vi "仪器参数设置.vi"(11 "仪器参数设置输入":T1(array[cluster])) -> (2 "确定":bool, 3 "仪器参数设置输出":T1(array[cluster]))   [LabVIEW 2016, in "斯坦道多参数.lvlib"]
uses:
  <vilib>/Utility/miscctls.llb/LVPointTypeDef.ctl
panel:
  in  "多参数":T2(ring)
  in  "标样校准时间":timestamp
  in  "二次多项式系数":dbl
  in  "线性相关系数":dbl
  in  "测量信号值":dbl
  in  "测量检出限":dbl
  in  "曲线斜率":dbl
  in  "曲线截距":dbl
  in  "空白校准时间":timestamp
  in  "消解时长":dbl
  in  "消解温度":dbl
  in  "测量间隔":dbl
  in  "测量精度":dbl
  in  "测量量程":dbl
  in  "取消":bool
  in  "确定":bool
  # "仪器参数设置"
  # "多参数"
  # "监测参数"
  # "黑色框参数需要手动输入\n灰色框参数自动读取不需要手动输入"
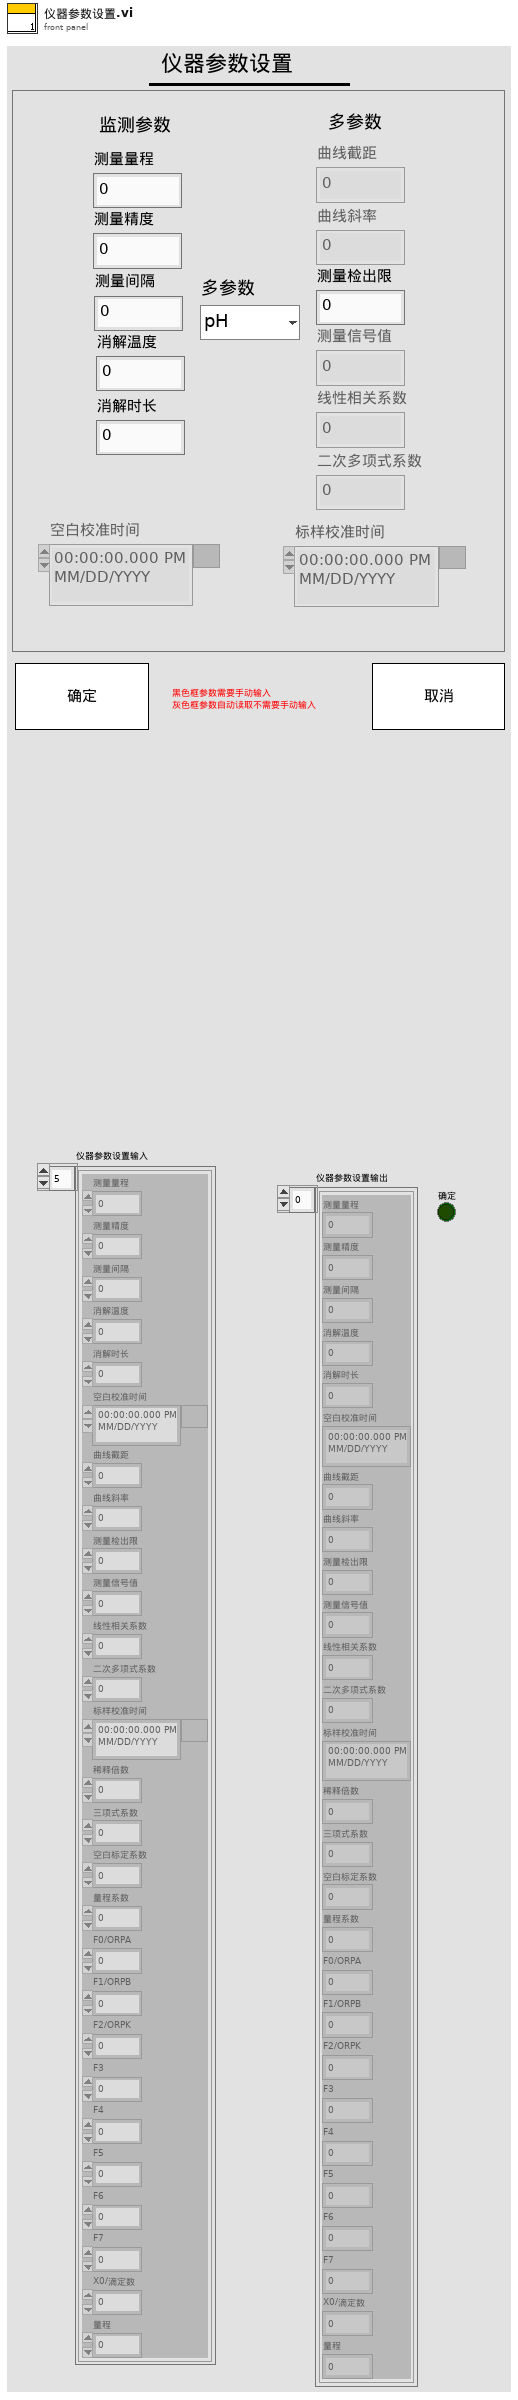
[diagram p1: front panel]
types:
  T1 = cluster{"测量量程":dbl, "测量精度":dbl, "测量间隔":dbl, "消解温度":dbl, "消解时长":dbl, "空白校准时间":timestamp, "曲线截距":dbl, "曲线斜率":dbl, "测量检出限":dbl, "测量信号值":dbl, "线性相关系数":dbl, "二次多项式系数":dbl, "标样校准时间":timestamp, "稀释倍数":dbl, "三项式系数":dbl, "空白标定系数":dbl, "量程系数":dbl, "F0/ORPA":dbl, "F1/ORPB":dbl, "F2/ORPK":dbl, "F3":dbl, "F4":dbl, "F5":dbl, "F6":dbl, "F7":dbl, "X0/滴定数":dbl, "量程":dbl}[]
  T2 = enum16{"pH", "水温", "电导率", "溶解氧", "浊度", "叶绿素", "藻密度", "ORP"}
  T3 = typedef "LVPointTypeDef.ctl" = cluster{"Horizontal":i16, "Vertical":i16}
  T4 = cluster{"测量量程":dbl, "测量精度":dbl, "测量间隔":dbl, "消解温度":dbl, "消解时长":dbl, "空白校准时间":timestamp, "曲线截距":dbl, "曲线斜率":dbl, "测量检出限":dbl, "测量信号值":dbl, "线性相关系数":dbl, "二次多项式系数":dbl, "标样校准时间":timestamp, "稀释倍数":dbl, "三项式系数":dbl, "空白标定系数":dbl, "量程系数":dbl, "F0/ORPA":dbl, "F1/ORPB":dbl, "F2/ORPK":dbl, "F3":dbl, "F4":dbl, "F5":dbl, "F6":dbl, "F7":dbl, "X0/滴定数":dbl, "量程":dbl}
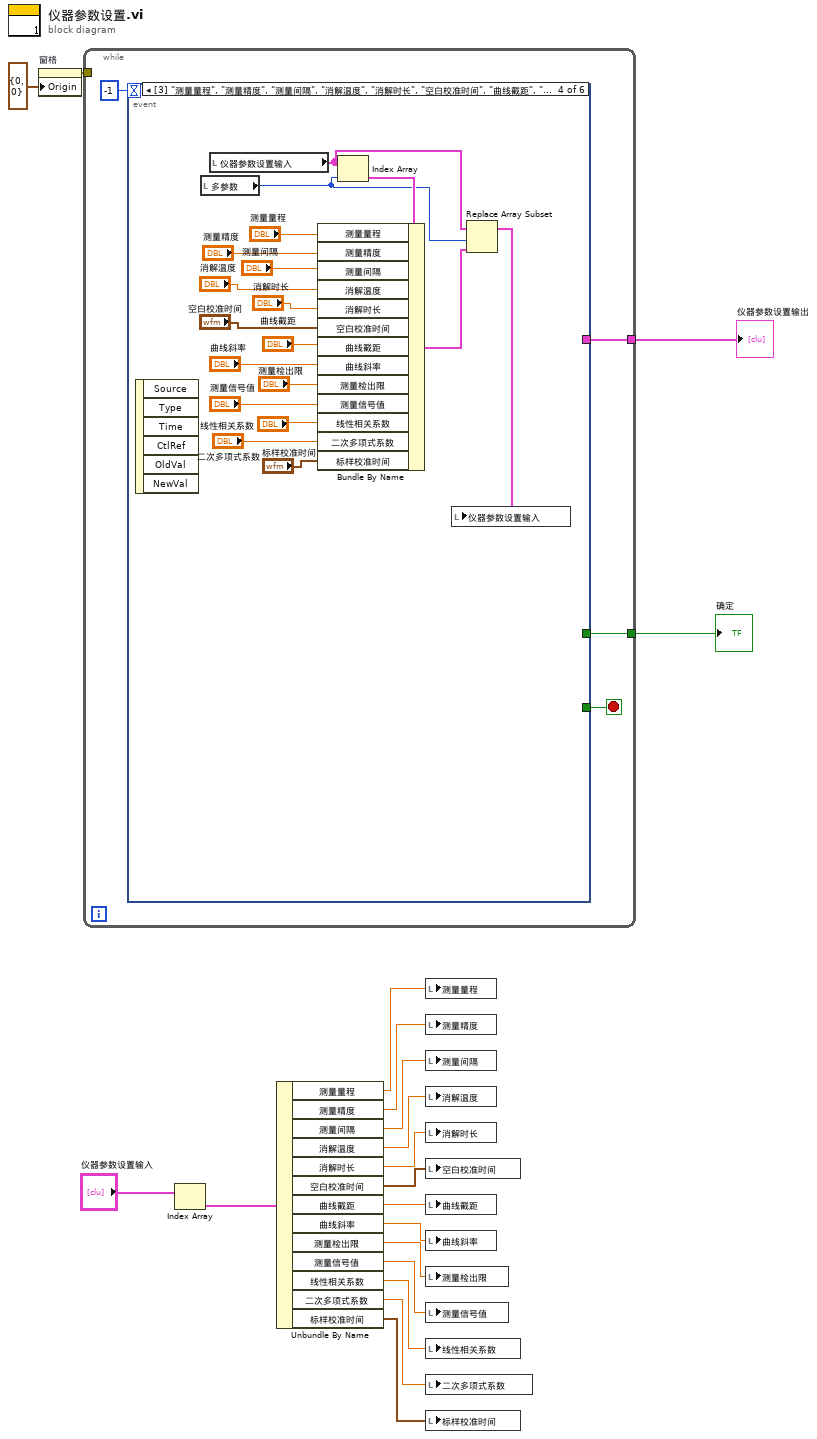
[diagram p0: block diagram]
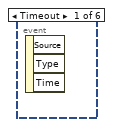
[diagram p2: hidden frame]
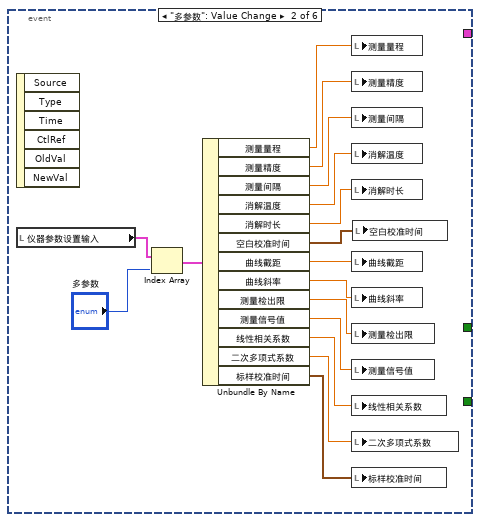
[diagram p3: hidden frame]
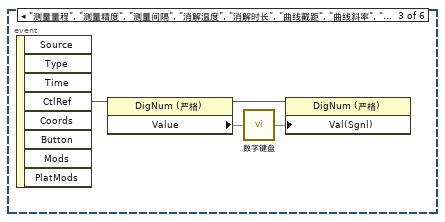
[diagram p4: hidden frame]
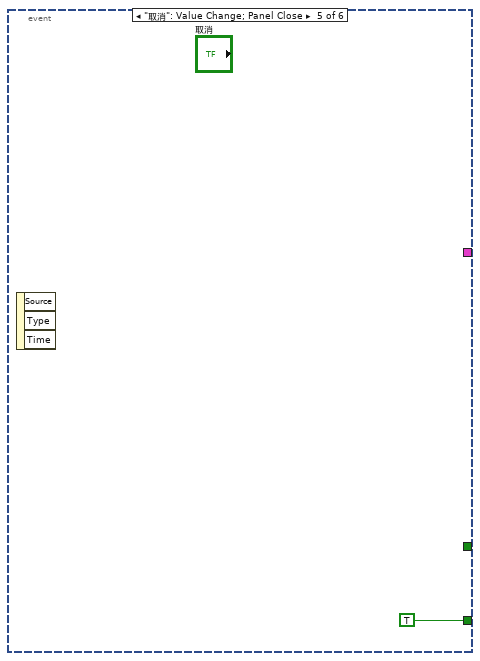
[diagram p5: hidden frame]
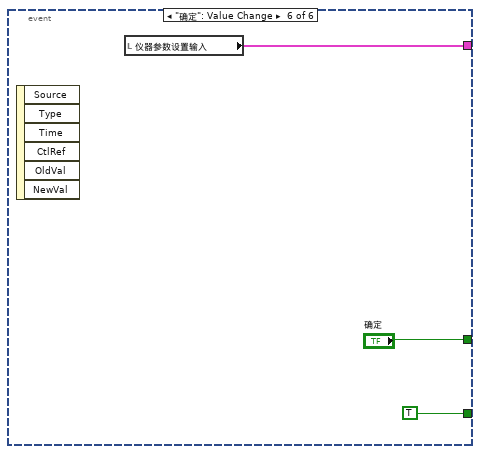
[diagram p6: hidden frame]
diagram:
  n1 = property on="窗格" class="Pane"("Origin"=T3 {"Horizontal"=0, "Vertical"=0} ("原点")) -> (error out=w18:errorcluster)  [unwired: 2 in, 1 out]
  n2 = while {
    tunnel: w18 -> [_]
    tunnel: [w22] -> w2
    tunnel: [w21] -> w1
    stop <- w23 stop-if-true
    n3 = event shown="[3] \"测量量程\", \"测量精度\", \"测量间隔\", \"消解温度\", \"消解时长\", \"空白校准时间\", \"曲线截距\", \"曲线斜率\", \"测量检出限\", \"测量信号值\", \"线性相关系数\", \"二次多项式系数\", \"标样校准时间\": 值改变" {
      selector: _ -> [_ _ _ _ _ _]
      dyn-events: _ -> [_ _ _ _ _ _]
      timeout: -1 -> [_ _ _ _ _ _]
      tunnel: [_ _ _ _ TRUE TRUE] -> w23
      tunnel: [_ _ _ _ _ "确定"] -> w22
      tunnel: [_ _ _ _ _ w63] -> w21
      event Timeout {
        n4 = event-data() -> ()  [unwired: 1 in, 3 out]
      }
      event "多参数": Value Change {
        n5 = event-data() -> ()  [unwired: 1 in, 6 out]
        n6 = local read "仪器参数设置输入"() -> (w25:T1)
        n7 = Index Array(array=w25, index="多参数") -> (element=w39:T4)
        n8 = Unbundle By Name(w39) -> ("测量量程"=w26:dbl, "测量精度"=w27:dbl, "测量间隔"=w28:dbl, "消解温度"=w29:dbl, "消解时长"=w30:dbl, "空白校准时间"=w31:timestamp, "曲线截距"=w32:dbl, "曲线斜率"=w33:dbl, "测量检出限"=w34:dbl, "测量信号值"=w35:dbl, "线性相关系数"=w36:dbl, "二次多项式系数"=w37:dbl, "标样校准时间"=w38:timestamp)
        n9 = local write "测量量程"(w26) -> ()
        n10 = local write "测量精度"(w27) -> ()
        n11 = local write "测量间隔"(w28) -> ()
        n12 = local write "消解温度"(w29) -> ()
        n13 = local write "消解时长"(w30) -> ()
        n14 = local write "曲线截距"(w32) -> ()
        n15 = local write "曲线斜率"(w33) -> ()
        n16 = local write "测量检出限"(w34) -> ()
        n17 = local write "测量信号值"(w35) -> ()
        n18 = local write "线性相关系数"(w36) -> ()
        n19 = local write "二次多项式系数"(w37) -> ()
        n20 = local write "标样校准时间"(w38) -> ()
        n21 = local write "空白校准时间"(w31) -> ()
      }
      event "测量量程", "测量精度", "测量间隔", "消解温度", "消解时长", "曲线截距", "曲线斜率", "测量检出限", "测量信号值", "线性相关系数", "二次多项式系数": Mouse Down {
        n22 = event-data() -> ("CtlRef"=w42:refnum<vi>)  [unwired: 1 in, 7 out]
        n23 = property class="DigNum (严格)"(reference=w42) -> (reference out=w43:refnum<vi>, "Value"=w40:dbl)  [unwired: 1 in, 1 out]
        n24 = call "数字键盘.vi"("OldNumber"=w40) -> ("NewNumber"=w41:dbl)
        n25 = property class="DigNum (严格)"(reference=w43, "Val(Sgnl)"=w41) -> ()  [unwired: 1 in, 2 out]
      }
      event "测量量程", "测量精度", "测量间隔", "消解温度", "消解时长", "空白校准时间", "曲线截距", "曲线斜率", "测量检出限", "测量信号值", "线性相关系数", "二次多项式系数", "标样校准时间": Value Change {
        n26 = event-data() -> ()  [unwired: 1 in, 6 out]
        n27 = local read "多参数"() -> (w59:T2)
        n28 = local read "仪器参数设置输入"() -> (w60:T1)
        n29 = Index Array(array=w60, index=w59) -> (element=w61:T4)
        n30 = Bundle By Name(cluster=w61, "测量量程"="测量量程", "测量精度"="测量精度", "测量间隔"="测量间隔", "消解温度"="消解温度", "消解时长"="消解时长", "空白校准时间"="空白校准时间", "曲线截距"="曲线截距", "曲线斜率"="曲线斜率", "测量检出限"="测量检出限", "测量信号值"="测量信号值", "线性相关系数"="线性相关系数", "二次多项式系数"="二次多项式系数", "标样校准时间"="标样校准时间") -> (w58:T4)
        n31 = Replace Array Subset(array=w60, new element=w58, index=w59) -> (w57:T1)
        n32 = local write "仪器参数设置输入"(w57) -> ()
      }
      event "取消": Value Change; Panel Close {
        n33 = event-data() -> ()  [unwired: 1 in, 3 out]
      }
      event "确定": Value Change {
        n34 = event-data() -> ()  [unwired: 1 in, 6 out]
        n35 = local read "仪器参数设置输入"() -> (w63:T1)
      }
    }
  }
  "仪器参数设置输出" <- w1
  "确定" <- w2
  n36 = Index Array(array="仪器参数设置输入") -> (element=w3:T4)  [unwired: 1 in]
  n37 = Unbundle By Name(w3) -> ("测量量程"=w17:dbl, "测量精度"=w16:dbl, "测量间隔"=w15:dbl, "消解温度"=w14:dbl, "消解时长"=w13:dbl, "空白校准时间"=w12:timestamp, "曲线截距"=w11:dbl, "曲线斜率"=w10:dbl, "测量检出限"=w9:dbl, "测量信号值"=w8:dbl, "线性相关系数"=w7:dbl, "二次多项式系数"=w6:dbl, "标样校准时间"=w5:timestamp)
  n38 = local write "测量量程"(w17) -> ()
  n39 = local write "测量精度"(w16) -> ()
  n40 = local write "测量间隔"(w15) -> ()
  n41 = local write "消解温度"(w14) -> ()
  n42 = local write "消解时长"(w13) -> ()
  n43 = local write "空白校准时间"(w12) -> ()
  n44 = local write "曲线截距"(w11) -> ()
  n45 = local write "曲线斜率"(w10) -> ()
  n46 = local write "测量检出限"(w9) -> ()
  n47 = local write "测量信号值"(w8) -> ()
  n48 = local write "线性相关系数"(w7) -> ()
  n49 = local write "二次多项式系数"(w6) -> ()
  n50 = local write "标样校准时间"(w5) -> ()
